vi "Authenticate.vi"(5 "Username":string, 7 "Address":string, 8 "Error In":errorcluster) -> (0 "Error Out":errorcluster)   [LabVIEW 2018, in "Tests.lvlib" / "Agent.lvlib"]
uses:
  Agent.lvlib
  <vilib>/addons/_JKI Toolkits/Caraya/classes/Test/Test.lvclass
  <vilib>/addons/_JKI Toolkits/Caraya/classes/Assert/Assert.lvclass
  src/Toolkit/Agent/Agent.lvclass
  src/Toolkit/Agent Identity/Agent Identity.lvclass
  src/Toolkit/SSH/SSH.lvclass
  src/Toolkit/Session/Session.lvclass
  Tests.lvlib
  src/Toolkit/Agent Identity/Support/Create from Agent.vi
  src/Toolkit/Agent/Support/Create from Session.vi
  src/Toolkit/Agent Identity/Support/Destroy to Agent.vi
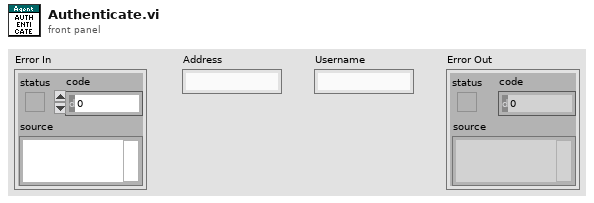
[diagram p1: front panel]
types:
  T1 = typedef "Toolkit.lvlib/Agent.lvclass/Results.ctl" = i32
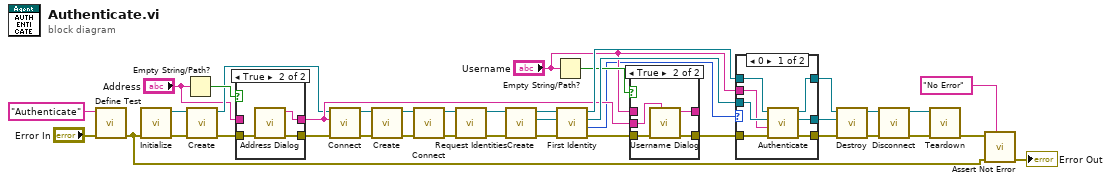
[diagram p0: block diagram]
diagram:
  n1 = call <vilib>:"Define Test.vi"("error in (no error)"="Error In", "Label (VI Title)"="Authenticate") -> ("error out"=w1:errorcluster)  [unwired: 9 in]
  n2 = call "Initialize.vi"("Error In"=w1) -> ("Error Out"=w11:errorcluster, "SSH"=w12:refnum<class "SSH.lvclass">)  [unwired: 9 in]
  n3 = Empty String/Path?(string/path="Address") -> (empty?=w14:bool)
  n4 = call "Create.vi"("Error In"=w11, "SSH"=w12) -> ("Error Out"=w15:errorcluster, "Sesssion"=w13:refnum<class "Session.lvclass">)  [unwired: 8 in]
  n5 = case shown="True" w14 {
    tunnel: w15 -> [w40 w44]
    tunnel: [w40 w43] -> w16
    tunnel: [w41 w42] -> w18
    tunnel: "Address" -> [w41 _]
    frame False {
    }
    frame True {
      n6 = call "Address Dialog.vi"("Error In"=w44) -> ("Error Out"=w43:errorcluster, "Address Out"=w42:string)  [unwired: 9 in]
    }
  }
  n7 = call "Connect.vi"("Error In"=w16, "Address"=w18, "Session In"=w13) -> ("Error Out"=w6:errorcluster, "Sesssion Out"=w10:refnum<class "Session.lvclass">)  [unwired: 7 in]
  n8 = call-poly "Create.vi"("Error In"=w6, "Session"=w10) -> ("Error Out"=w8:errorcluster, "Agent"=w9:refnum<class "Agent.lvclass">)  [unwired: 8 in]
  n9 = call "Connect.vi"("Error In"=w8, "Agent In"=w9) -> ("Error Out"=w35:errorcluster, "Agent Out"=w36:refnum<class "Agent.lvclass">)  [unwired: 8 in]
  n10 = call "Request Identities.vi"("Error In"=w35, "Agent In"=w36) -> ("Error Out"=w33:errorcluster, "Agent Out"=w34:refnum<class "Agent.lvclass">)  [unwired: 8 in]
  n11 = call-poly "Create.vi"("Error In"=w33, "Agent In"=w34) -> ("Error Out"=w31:errorcluster, "Identity"=w30:refnum<class "Agent Identity.lvclass">, "Agent Out"=w32:refnum<class "Agent.lvclass">)  [unwired: 7 in]
  n12 = Empty String/Path?(string/path="Username") -> (empty?=w17:bool)
  n13 = call "First Identity.vi"("Error In"=w31, "Identity In"=w30, "Agent In"=w32) -> ("Error Out"=w5:errorcluster, "Result"=w2:T1, "Identity Out"=w19:refnum<class "Agent Identity.lvclass">, "Agent Out"=w20:refnum<class "Agent.lvclass">)  [unwired: 5 in]
  n14 = case shown="True" w17 {
    tunnel: w5 -> [w46 w50]
    tunnel: [w45 w49] -> _
    tunnel: [w46 w48] -> w4
    tunnel: "Username" -> [w45 _]
    tunnel: w18 -> [_ w47]
    frame False {
    }
    frame True {
      n15 = call "Username Dialog.vi"("Address"=w47, "Error In"=w50) -> ("Error Out"=w48:errorcluster, "Username Out"=w49:string)  [unwired: 8 in]
    }
  }
  n16 = case shown="0" w2 {
    tunnel: [w57 w58] -> w23
    tunnel: [w56 w60] -> w22
    tunnel: [w55 w59] -> w21
    tunnel: w20 -> [w54 w60]
    tunnel: w19 -> [w53 w59]
    tunnel: "Username" -> [w52 _]
    tunnel: w4 -> [w51 w58]
    frame 0 {
      n17 = call "Authenticate.vi"("Error In"=w51, "Username"=w52, "Identity In"=w53, "Agent In"=w54) -> ("Error Out"=w57:errorcluster, "Identity Out"=w55:refnum<class "Agent Identity.lvclass">, "Agent Out"=w56:refnum<class "Agent.lvclass">)  [unwired: 5 in]
    }
    frame 1 {
    }
  }
  n18 = call-poly "Destroy.vi"("Error In"=w23, "Identity"=w21, "Agent In"=w22) -> ("Error Out"=w27:errorcluster, "Agent Out"=w28:refnum<class "Agent.lvclass">)  [unwired: 7 in]
  n19 = call "Disconnect.vi"("Error In"=w27, "Agent In"=w28) -> ("Error Out"=w26:errorcluster, "Agent Out"=w25:refnum<class "Agent.lvclass">)  [unwired: 8 in]
  n20 = call "Teardown.vi"("Error In"=w26, "Agent"=w25) -> ("Error Out"=w29:errorcluster)  [unwired: 9 in]
  n21 = call <vilib>:"Assert Not Error.vi"("Label"="No Error", "error in (no error)"=w1, "Not Error?"=w29) -> ("error out"=→"Error Out":errorcluster)  [unwired: 8 in]
